vi "From File.vi"(7 "Set path to Paths? [T]":bool=TRUE, 8 "error in (no error)":errorcluster, 10 "Path":path, 11 "Carya Config in":refnum<class "Carya Config.lvclass">) -> (0 "error out":errorcluster, 3 "Carya Config out":refnum<class "Carya Config.lvclass">)   [LabVIEW 2013, in "Carya Config.lvclass"]
doc: "Copyright 2018, Carya Automatisering, Wiebe Walstra."
uses:
  Carya Config.lvclass
  Carya Config.lvclass/Carya Config.ctl
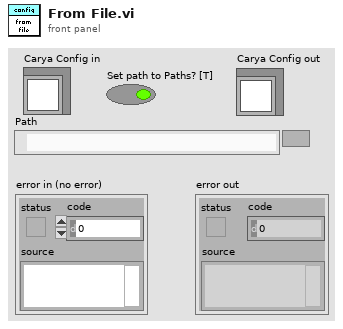
[diagram p1: front panel]
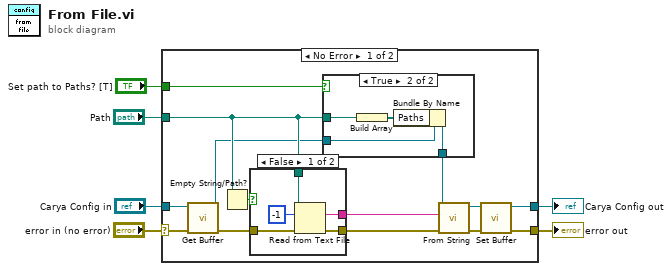
[diagram p0: block diagram]
diagram:
  n1 = case shown="No Error" "error in (no error)" {
    selector: "error in (no error)" -> [w19 w33]
    tunnel: [w13 w33] -> w5
    tunnel: [w12 w32] -> w4
    tunnel: "Path" -> [w15 _]
    tunnel: "Carya Config in" -> [w10 w32]
    tunnel: "Set path to Paths? [T]" -> [w7 _]
    frame No Error {
      n2 = call-dynamic "Get Buffer.vi"("error in (no error)"=w19, "Carya Config in"=w10) -> ("error out"=w11:errorcluster, "Config"=w8:refnum<class "Carya Config.lvclass">)  [unwired: 8 in]
      n3 = Empty String/Path?(string/path=w15) -> (empty?=w16:bool)
      n4 = case shown="False" w16 {
        tunnel: w11 -> [w30 w31]
        tunnel: [w29 w31] -> w18
        tunnel: w15 -> [w28 _]
        tunnel: [w27 _] -> w17
        frame False {
          n5 = Read from Text File(file (use dialog)=w28, count=-1, error in=w30) -> (text=w27:string, error out=w29:errorcluster)  [unwired: 1 in, 2 out]
        }
        frame True {
        }
      }
      n6 = case shown="True" w7 {
        tunnel: w15 -> [_ w25]
        tunnel: [w21 w24] -> w14
        tunnel: w8 -> [w21 w23]
        frame False {
        }
        frame True {
          n7 = Build Array(w25) -> (w22:path[])
          n8 = Bundle By Name(cluster=w23, "Paths"=w22) -> (w24:refnum<class "Carya Config.lvclass">)
        }
      }
      n9 = call-dynamic "From String.vi"("error in (no error)"=w18, "String"=w17, "Carya Config in"=w14) -> ("error out"=w20:errorcluster, "Carya Config out"=w9:refnum<class "Carya Config.lvclass">)  [unwired: 6 in, 1 out]
      n10 = call-dynamic "Set Buffer.vi"("error in (no error)"=w20, "Carya Config"=w9) -> ("error out"=w13:errorcluster, "Carya Config out"=w12:refnum<class "Carya Config.lvclass">)  [unwired: 8 in]
    }
    frame Error {
    }
  }
  "error out" <- w5
  "Carya Config out" <- w4
